vi "Keithley 648X Series Voltage Sweep Test.vi"() -> ()   [LabVIEW 2021]
doc: "This example shows how to configure a measurement and take multiple readings.\n\n<b>Note:</b>\nThis VI is only valid for Keithley 6487."
uses:
  <instrlib>/Keithley 648X Series/Keithley 648X Series.lvlib
panel:
  in  "Difficulty Class":enum32{"Easy", "Medium"}(tab)
  in  "Arm Loop Count":i32=1
  in  "Arm Source":u16(ring) items=["Immediate", "Timer", "Bus", "Tlink", "Manual", "Negative SOT", "Positive SOT", "Bidirectional SOT"]
  in  "Arm Timer Interval":dbl=0.1
  in  "Enable Arm Bypass":bool
  in  "Enable Trigger Bypass":bool
  in  "Trigger Delay":dbl
  in  "Trigger Loop Count":i32=1
  in  "Trigger Source":u16(ring) items=["Immediate", "Tlink"]
  in  "Voltage Sweep Step Size":dbl=1.0
  in  "Voltage Sweep Stop":dbl=10.0
  in  "Voltage Sweep Start":dbl
  in  "Voltage Sweep Delay":dbl=1.0
  out "Voltage Sweep Results":cluster{dbl[], dbl[]}(graph)
  in  "Serial Configuration":T1={"Baud Rate"=9600, "Parity"=0, "Data Bits"=8, "Stop Bits"=10, "Flow Control"=0} {"Flow Control" items=["None", "XON/XOFF", "RTS/CTS", "XON/XOFF & RTS/CTS", "DTR/DSR", "XON/XOFF & DTR/DSR"]; "Stop Bits" items=["1.0"=10, "1.5"=15, "2.0"=20]; "Data Bits" items=["7"=7, "8"=8]; "Parity" items=["None", "Odd", "Even", "Mark", "Space"]; "Baud Rate" items=["300"=300, "600"=600, "1200"=1200, "2400"=2400, "4800"=4800, "9600"=9600, "19200"=19200]}
  in  "VISA resource name":refnum<visa-resource-name>
  # "(c) 2017 National Instruments.  ALL RIGHTS RESERVED."
  # "Sweep Settings"
  # "Configure the Sweep Settings, and the Serial Configuration if need be. Then hit the run button."
  # "Make sure that the instrument is triggered for each of the voltage measurements in the sweep. Otherwise the sweep won't execute, or it executes, but the instrument does not function as expected."
  # "Also Make sure to configure the arm and trigger layers appropriately. The Read Sweep Results relies on\na wait loop that may never terminate if the configuration is not conducive to its termination."
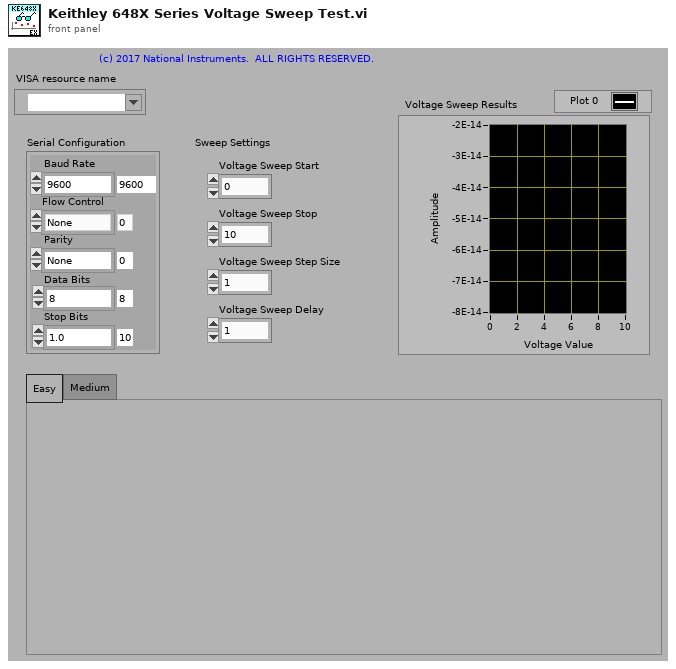
[diagram p1: front panel]
types:
  T1 = cluster{"Baud Rate":u32, "Parity":u16, "Data Bits":u16, "Stop Bits":u16, "Flow Control":u16}
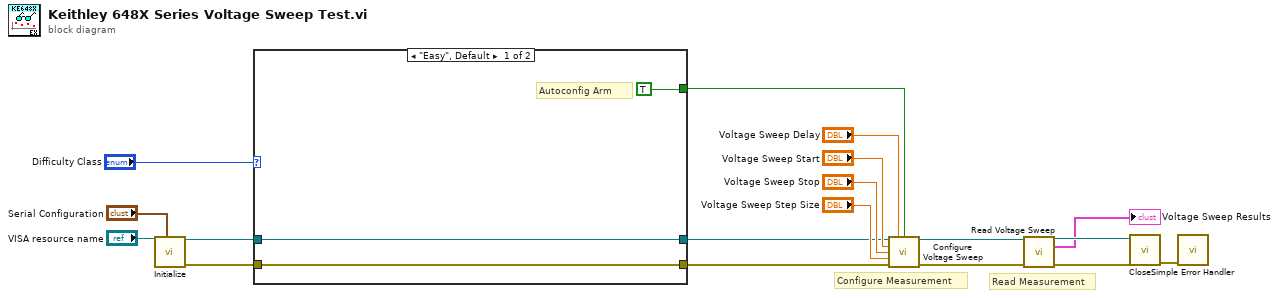
[diagram p0: block diagram]
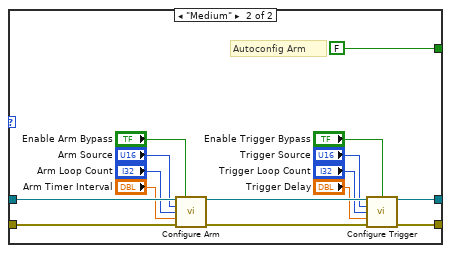
[diagram p2: hidden frame]
diagram:
  # "Read Measurement"
  # "Configure Measurement"
  n1 = call <instrlib>:"Initialize.vi"("Serial Configuration"="Serial Configuration", "VISA resource name"="VISA resource name") -> ("error out"=w3:errorcluster, "VISA resource name out"=w6:refnum<visa-resource-name>)  [unwired: 8 in]
  n2 = case shown="\"Easy\", Default" "Difficulty Class" {
    tunnel: [w21 w30] -> w5
    tunnel: w6 -> [w21 w35]
    tunnel: w3 -> [w20 w34]
    tunnel: [w20 w32] -> w4
    tunnel: [TRUE FALSE] -> w1
    frame "Easy", Default {
      # "Autoconfig Arm"
    }
    frame "Medium" {
      # "Autoconfig Arm"
      n3 = call <instrlib>:"Configure Arm.vi"("VISA resource name"=w35, "Enable Arm Bypass (F: Disable)"="Enable Arm Bypass", "Arm Source (0: Immediate)"="Arm Source", "Arm Loop Count (1)"="Arm Loop Count", "Arm Timer Interval (0.1 s)"="Arm Timer Interval", "error in (no error)"=w34) -> ("VISA resource name out"=w31:refnum<visa-resource-name>, "error out"=w33:errorcluster)  [unwired: 8 in]
      n4 = call <instrlib>:"Configure Trigger.vi"("VISA resource name"=w31, "Enable Trigger Bypass (F: Disable)"="Enable Trigger Bypass", "Trigger Source (0: Immediate)"="Trigger Source", "Trigger Loop Count (1)"="Trigger Loop Count", "Trigger Delay (0 s)"="Trigger Delay", "error in (no error)"=w33) -> ("VISA resource name out"=w30:refnum<visa-resource-name>, "error out"=w32:errorcluster)  [unwired: 8 in]
    }
  }
  n5 = call <instrlib>:"Configure Voltage Sweep.vi"("VISA resource name"=w5, "Voltage Sweep Delay (1s)"="Voltage Sweep Delay", "Autoconfig Arm (T: Enable)"=w1, "Voltage Sweep Start (0V)"="Voltage Sweep Start", "Voltage Sweep Stop (10V)"="Voltage Sweep Stop", "Voltage Sweep Step Size (1V)"="Voltage Sweep Step Size", "error in (no error)"=w4) -> ("VISA resource name out"=w12:refnum<visa-resource-name>, "error out"=w11:errorcluster)  [unwired: 7 in]
  n6 = call <instrlib>:"Read Voltage Sweep.vi"("VISA resource name"=w12, "error in (no error)"=w11) -> ("VISA resource name out"=w14:refnum<visa-resource-name>, "Voltage Sweep Results"=→"Voltage Sweep Results":cluster{dbl[], dbl[]}, "error out"=w15:errorcluster)  [unwired: 11 in]
  n7 = call <instrlib>:"Close.vi"("error in (no error)"=w15, "VISA resource name"=w14) -> ("error out"=w18:errorcluster)  [unwired: 9 in]
  n8 = call <vilib>:"Simple Error Handler.vi"("error in (no error)"=w18) -> ()  [unwired: 4 in, 5 out]
